vi "removeNode.vi"(0 "reference":refnum<class "CallNode.lvclass">, 1 "graph":refnum<class "Graph.lvclass">, 2 "node":refnum<class "AbstractNode.lvclass">, 5 "error in (no error)":errorcluster) -> (14 "reference out":refnum<class "CallNode.lvclass">, 19 "error out":errorcluster)   [LabVIEW 2020, in "CallNode.lvclass"]
uses:
  <resource>/Framework/Providers/Open_GDS/UML/CallNode_class/CallNode.lvclass
  C:/Program Files (x86)/National Instruments/LabVIEW 2020/resource/Framework/Providers/Open_GDS/UML/AbstractNode_class/AbstractNode.lvclass
  <resource>/Framework/Providers/Open_GDS/UML/AbstractNode_class/AbstractNode.lvclass
  <resource>/Framework/Providers/Open_GDS/UML/Graph_class/Graph.lvclass
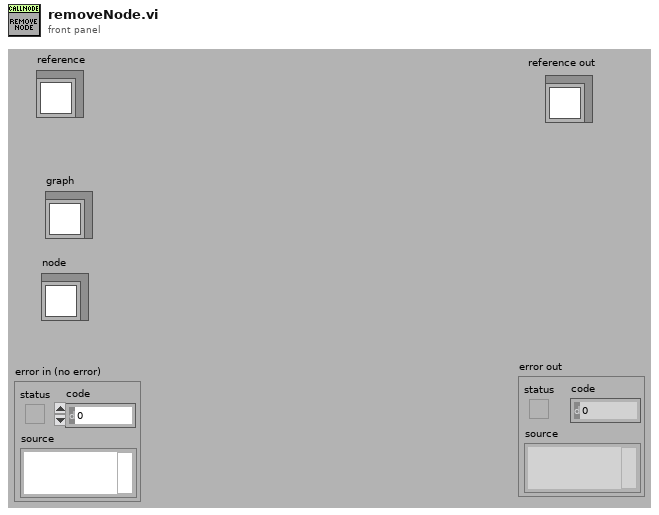
[diagram p1: front panel]
types:
  T1 = typedef "CallNode.lvclass/ObjectAttributes.ctl" = cluster{"objectCallNodeRef":refnum<class "AbstractNode.lvclass">, "signaled":bool, "openBottom":bool, "DEFAULT_WIDTH":i32, "DEFAULT_HEIGHT":i32, "CALL_YGAP":i32}
  T2 = typedef "AbstractNode.lvclass/ObjectAttributes.ctl" = cluster{"parent":refnum<class "AbstractNode.lvclass">, "children":refnum<class "AbstractNode.lvclass">[], "Hidden":bool}
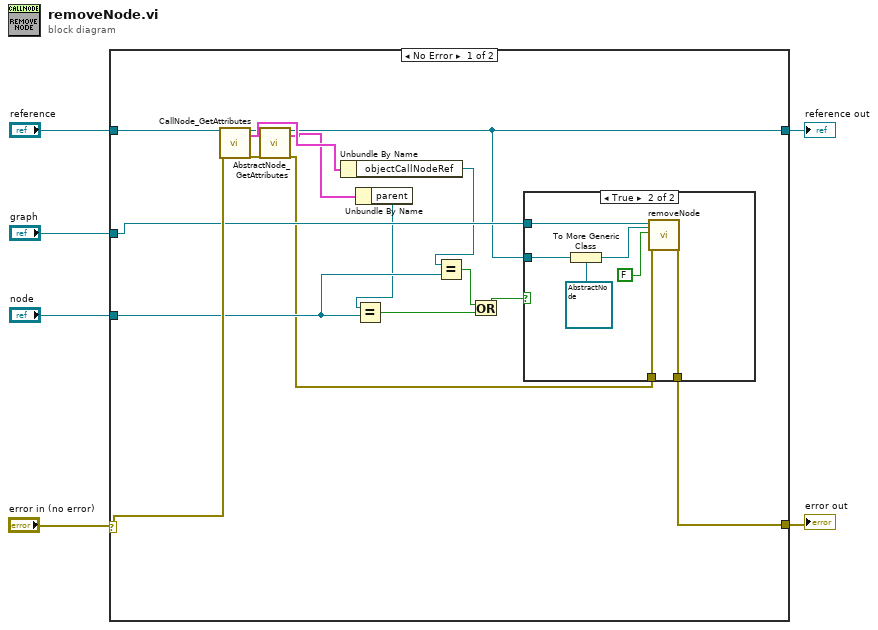
[diagram p0: block diagram]
diagram:
  n1 = case shown="No Error" "error in (no error)" {
    selector: "error in (no error)" -> [w20 w31]
    tunnel: "reference" -> [w22 w32]
    tunnel: [w21 w31] -> w5
    tunnel: [w8 w32] -> w4
    tunnel: "graph" -> [w19 _]
    tunnel: "node" -> [w18 _]
    frame No Error {
      n2 = call <resource>:"CallNode_GetAttributes.vi"("reference in"=w22, "error in (no error)"=w20) -> ("reference out"=w11:refnum<class "CallNode.lvclass">, "Data"=w12:T1, "error out"=w10:errorcluster)  [unwired: 1 in, 14 out]
      n3 = call <resource>:"AbstractNode_GetAttributes.vi"("reference in"=w11, "error in (no error)"=w10) -> ("reference out"=w8:refnum<class "CallNode.lvclass">, "Data"=w7:T2, "error out"=w9:errorcluster)  [unwired: 14 in, 1 out]
      n4 = Unbundle By Name(w12) -> ("objectCallNodeRef"=w16:refnum<class "AbstractNode.lvclass">)
      n5 = Unbundle By Name(w7) -> ("parent"=w17:refnum<class "AbstractNode.lvclass">)
      n6 = Equal?(x=w17, y=w18) -> (x = y?=w15:bool)
      n7 = Equal?(x=w16, y=w18) -> (x = y?=w14:bool)
      n8 = Or(x=w14, y=w15) -> (x .or. y?=w13:bool)
      n9 = case shown="True" w13 {
        tunnel: w19 -> [_ w30]
        tunnel: w9 -> [w23 w29]
        tunnel: [w23 w28] -> w21
        tunnel: w8 -> [_ w27]
        frame False {
        }
        frame True {
          n10 = To More Generic Class(target class=refnum<class "AbstractNode.lvclass"> refnum ("node"), reference=w27) -> (generic class reference=w25:refnum<class "AbstractNode.lvclass">)
          n11 = call-dynamic "removeNode.vi"("reference"=w30, "node"=w25, "RemoveChildrenIfAny(False)"=FALSE, "error in (no error)"=w29) -> ("error out"=w28:errorcluster)  [unwired: 14 in, 1 out]
        }
      }
    }
    frame Error {
    }
  }
  "reference out" <- w4
  "error out" <- w5
